vi "Result_Test.vi"(8 "error in (no error)":errorcluster caption="entrée d'erreur (pas d'erreur)", 11 "Get_Voltage en entrée":refnum<class "Nodon_Get_HW_Version.lvclass">) -> (0 "error out":errorcluster caption="sortie d'erreur", 3 "Get_Voltage en sortie":refnum<class "Nodon_Get_HW_Version.lvclass">)   [LabVIEW 2020, in "Library Test.lvlib" / "Nodon_Get_HW_Version.lvclass"]
uses:
  Nodon_Get_HW_Version.lvclass
  C:/Users/ngarcin/OneDrive - Altyor/Standard TB/Suite TB45/Class/Test/Test (Default)/Test (Default).lvclass
  Commun VI/TypeDef/Variable Printable.ctl
  JSON API/JSON Value/Set from JSON string.vi
  JSON API/JSON Value/JSON Value.lvclass
  Nodon_Send_Command_UART.lvclass
  JSON API/Variant JSON/Variant JSON.lvlib
  JSON API/Get Polymorphic/JSON GetSet.lvlib
  Commun VI/Library Commun.lvlib
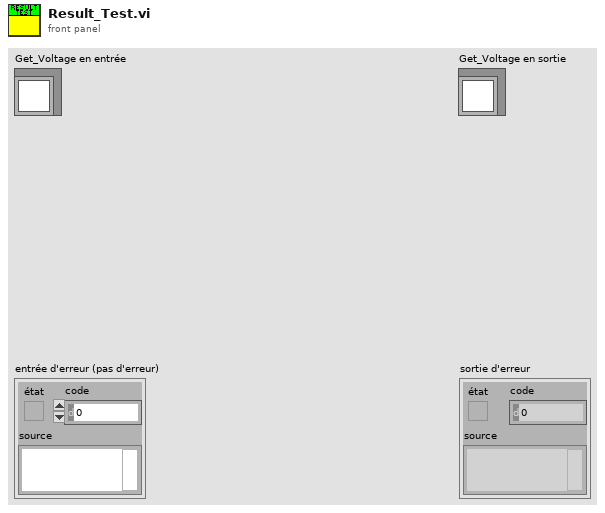
[diagram p1: front panel]
types:
  T1 = typedef "Variable Printable.ctl" = string
  T2 = enum16{"Get Variable", "Get All Variables", "Set Variable", "Delete Variable", "Delete All Variable"}
  T3 = cluster{"Commande Type":string, "Command ID":string, "Data":string, "Error":string}
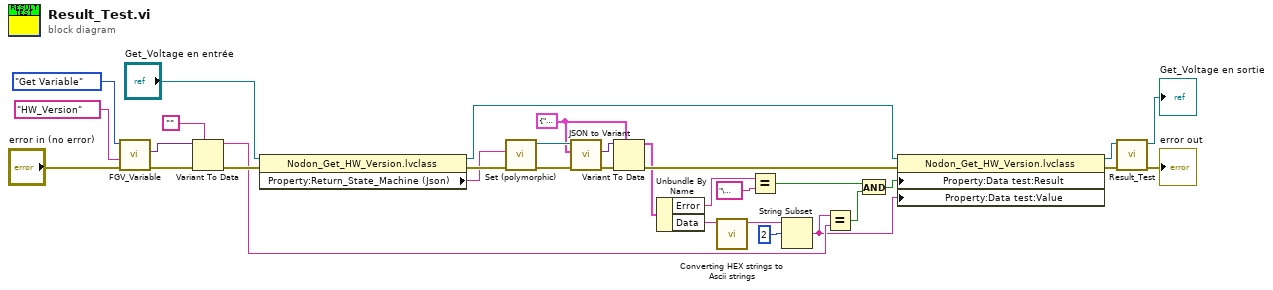
[diagram p0: block diagram]
diagram:
  w17 = T3 {"Commande Type"="", "Command ID"="", "Data"="", "Error"=""}
  n1 = call "FGV_Variable.vi"("error in (no error)"="error in (no error)", "Variable"=T1 "HW_Version", "Function"=T2."Get Variable") -> ("error out"=w12:errorcluster, "Data Out"=w11:variant)  [unwired: 6 in, 1 out]
  n2 = Variant To Data(error in=w12, type="", Variant=w11) -> (data=w7:string, error out=w8:errorcluster)
  n3 = property class="Nodon_Get_HW_Version.lvclass"(reference="Get_Voltage en entrée", error in=w8) -> (reference out=w30:refnum<class "Nodon_Get_HW_Version.lvclass">, error out=w25:errorcluster, "Property:Return_State_Machine (Json)"=w23:string)
  n4 = call-poly "Set (polymorphic).vi"("error in (no error)"=w25, "JSON stream"=w23) -> ("error out"=w27:errorcluster, "JSON Value out"=w29:refnum<class "JSON Value.lvclass">)  [unwired: 7 in, 1 out]
  n5 = call "JSON to Variant.vi"("error in (no error)"=w27, "Variant (Data Type)"=w17, "JSON Value"=w29) -> ("error out"=w28:errorcluster, "Variant out"=w26:variant)  [unwired: 7 in]
  n6 = Variant To Data(error in=w28, type=w17, Variant=w26) -> (data=w22:T3, error out=w24:errorcluster)
  n7 = Unbundle By Name(w22) -> ("Error"=w21:string, "Data"=w15:string)
  n8 = call "Converting HEX strings to Ascii strings.vi"("chaîne IN"=w15) -> ("Chaîne OUT"=w2:string)  [unwired: 9 in, 1 out]
  n9 = Equal?(x=w21, y="\u0000") -> (x = y?=w5:bool)
  n10 = String Subset(string=w2, offset (0)=2) -> (substring=w1:string)  [unwired: 1 in]
  n11 = Equal?(x=w1, y=w7) -> (x = y?=w6:bool)
  n12 = And(x=w5, y=w6) -> (x .and. y?=w4:bool)
  n13 = property class="Nodon_Get_HW_Version.lvclass"(reference=w30, error in=w24, "Property:Data test:Result"=w4, "Property:Data test:Value"=w1) -> (reference out=w18:refnum<class "Nodon_Get_HW_Version.lvclass">, error out=w16:errorcluster)
  n14 = call-parent "Result_Test.vi"("error in (no error)"=w16, "Get_Voltage en entrée"=w18) -> ("error out"=→"error out":errorcluster, "Get_Voltage en sortie"=→"Get_Voltage en sortie":refnum<class "Nodon_Get_HW_Version.lvclass">)  [unwired: 8 in]
